vi "EEG_2022_040_LabView_3.1.vi"() -> ()   [LabVIEW 2022 SP3]
panel:
  out "Warning Text":string
  out "Warning?":bool
  in  "Min.  Temperature":dbl
  in  "Max.  Temperature":dbl
  in  "Current  Temperatue":dbl
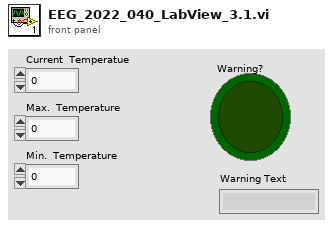
[diagram p1: front panel]
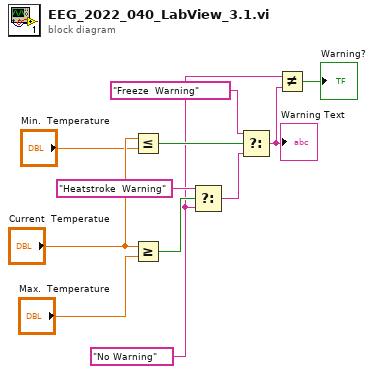
[diagram p0: block diagram]
diagram:
  w3 = "No Warning"
  n1 = Less Or Equal?(x="Current  Temperatue", y="Min.  Temperature") -> (x <= y?=w6:bool)
  n2 = Greater Or Equal?(x="Current  Temperatue", y="Max.  Temperature") -> (x >= y?=w8:bool)
  n3 = Select(t="Heatstroke  Warning", s=w8, f=w3) -> (s? t:f=w5:string)
  n4 = Select(t="Freeze  Warning", s=w6, f=w5) -> (s? t:f=w1:string)
  "Warning Text" <- w1
  n5 = Not Equal?(x=w3, y=w1) -> (x != y?=→"Warning?":bool)
